vi "overlayToPointList.vi"(1 "Overlay":cluster{"X":dbl, "Y":dbl, "Z":dbl}[](array[cluster])) -> (0 "PointList":dbl[][](array[numeric]))   [LabVIEW 2017]
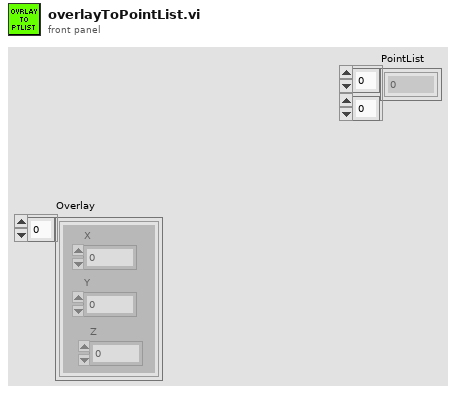
[diagram p1: front panel]
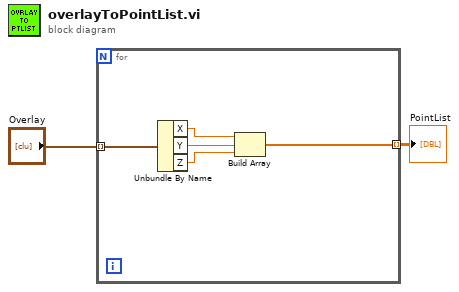
[diagram p0: block diagram]
diagram:
  n1 = for {
    tunnel: "Overlay" -> [w7] mode=indexing
    tunnel: [w3] -> w1 mode=indexing
    n2 = Unbundle By Name(w7) -> ("X"=w6:dbl, "Y"=w5:dbl, "Z"=w4:dbl)
    n3 = Build Array(w6, w5, w4) -> (w3:dbl[])
  }
  "PointList" <- w1
